vi "CreateAccessorFolder.vi"(8 "error in":errorcluster, 10 "Name":string, 11 "LabVIEW Class In":refnum<vi>) -> (0 "error out":errorcluster, 3 "LabVIEW Class Out":refnum<vi>)   [LabVIEW 2013, in "baseClass.lvclass"]
uses:
  baseClass.lvclass
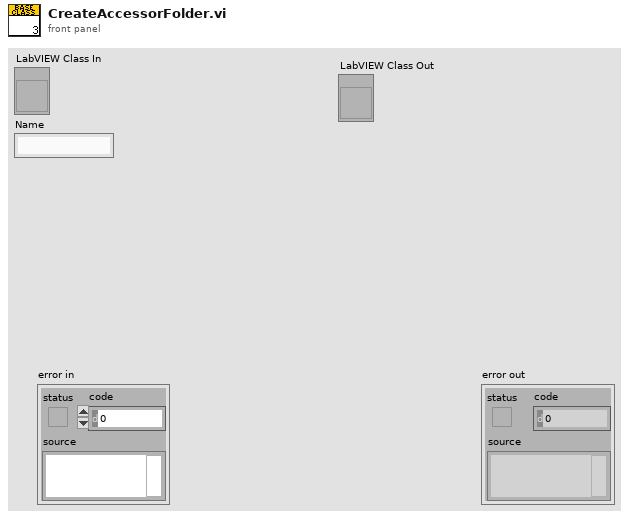
[diagram p1: front panel]
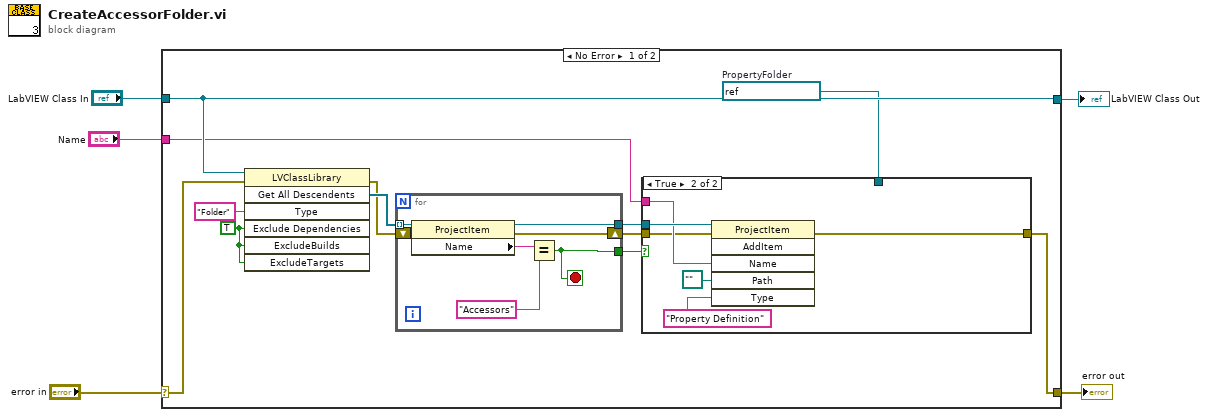
[diagram p0: block diagram]
diagram:
  n1 = case shown="No Error" "error in" {
    selector: "error in" -> [w9 w32]
    tunnel: [w7 w32] -> w4
    tunnel: "LabVIEW Class In" -> [w17 w31]
    tunnel: [w17 w31] -> w2
    tunnel: "Name" -> [w10 _]
    frame No Error {
      w6 = refnum<vi> refnum  # PropertyFolder
      w15 = TRUE ("ExcludeDependencies")
      n2 = invoke class="LVClassLibrary" method="Get All Descendents"(reference=w17, error in=w9, "Type"="Folder", "Exclude Dependencies"=w15, "ExcludeBuilds"=w15, "ExcludeTargets"=w15) -> (error out=w13:errorcluster, "All Descendents"=w14:refnum<vi>[])  [unwired: 1 in, 5 out]
      n3 = for {
        tunnel: w14 -> [w30] mode=indexing
        tunnel: [w27] -> w12
        tunnel: [w26] -> w11
        shift-right: [w25] -> w8
        shift-left: w13 -> [_]
        stop <- w27 stop-if-true
        n4 = property class="ProjectItem"(reference=w30) -> (reference out=w26:refnum<vi>, error out=w25:errorcluster, "Name"=w29:string)  [unwired: 1 in]
        n5 = Equal?(x=w29, y="Accessors") -> (x = y?=w27:bool)
      }
      n6 = case shown="True" w12 {
        tunnel: w11 -> [_ w24]
        tunnel: w10 -> [_ w23]
        tunnel: w8 -> [w18 w22]
        tunnel: [w18 w19] -> w7
        tunnel: w6 -> [_ _]
        frame False {
        }
        frame True {
          n7 = invoke class="ProjectItem" method="AddItem"(reference=w24, error in=w22, "Name"=w23, "Path"=path "", "Type"="Property Definition") -> (error out=w19:errorcluster)  [unwired: 1 in, 5 out]
        }
      }
    }
    frame Error {
    }
  }
  "error out" <- w4
  "LabVIEW Class Out" <- w2
